vi "MS4_demo.vi"() -> ()   [LabVIEW 2012]
uses:
  States.ctl
  <vilib>/vision/Image Controls.llb/IMAQ Image.ctl
  <vilib>/httpClient/ClientHandle.ctl
  <vilib>/Platform/TimedLoop/XDataNode/timing_clust.ctl
  <vilib>/Platform/TimedLoop/XDataNode/nitl_modes.ctl
  <vilib>/Platform/TimedLoop/XDataNode/wakeup.ctl
  <vilib>/FPGAPlugInAG/sbRIO-9636/niLvFpga_Open_sbRIO-9636.vi
  <vilib>/rvi/interface/common/dynamic/niFpgaDynamicAddResources.vi
  Globals.vi
  <vilib>/Utility/error.llb/Error Cluster From Error Code.vi
  <vilib>/rvi/errors/niLvFpgaAdjustHostInterfaceError.vi
  <vilib>/FPGAPlugInAG/Dynamic/niLvFpga_Close_Dynamic.vi
  <vilib>/platform/TimedLoop/XDataNode/XDataNode.xnode
  <vilib>/rvi/interface/nirviOpenFPGA/nirviOpenFPGA.xnode
  FPGA Bitfiles/NIARC_FPGATarget_FPGACompile_e4XhunWUay0.lvbitx
  <vilib>/rvi/interface/nirviReadWriteControl/nirviReadWriteControl.xnode
  <vilib>/rvi/interface/nirviCloseFPGA/nirviCloseFPGA.xnode
  <vilib>/Platform/TimedLoop/XDataNode/XDNodeRunTimeDep.lvlib
  <vilib>/httpClient/LabVIEWHTTPClient.lvlib
  NiFpgaLv.dll
  <vilib>/rvi/interface/Simulation/niFpgaSimulationCallBeginRW.vi
panel:
  in  "WaypointWaypoints 2":dbl[][](array[numeric])
  in  "WaypointWaypoints":dbl[][](array[numeric])
  in  "Go to block?":bool=TRUE
  out "Arm State":enum16{"arm down", "push", "turn", "arm up"}(ring)
  out "Current \nState":T1(ring)
  in  "Claw deadband":dbl=0.05
  in  "Block Claw distance":dbl=0.25
  in  "stop":bool
  in  "Enable":bool
  in  "Block Mid Range":dbl=50.0
  in  "Block X-Offset":dbl=100.0
  # "Ignore Front ir"
  # "Heading"
  # "Forward Speed"
  # "Time (ms)"
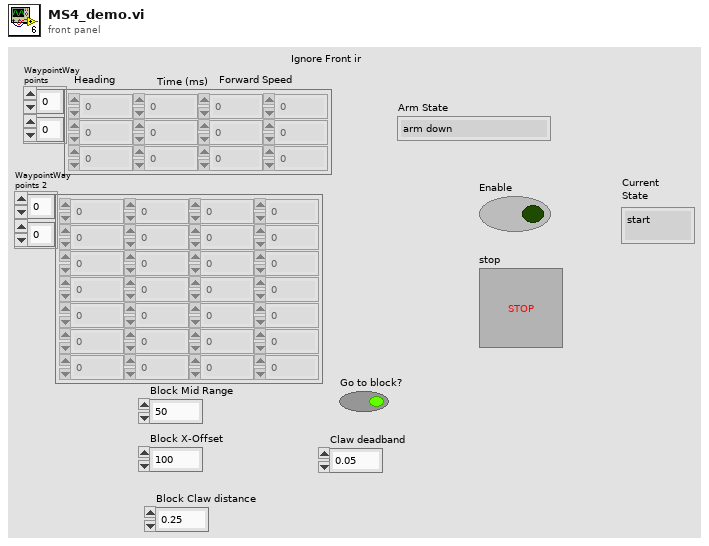
[diagram p1: front panel]
types:
  T1 = enum16{"start", "drive", "turning", "find block", "align block", "pickup"}
  T2 = cluster{"X Velocity (m/s)":dbl, "Y Velocity (m/s)":dbl, "Angular Velocity (rad/s)":dbl}
  T3 = typedef "IMAQ Image.ctl" = refnum<image>
  T4 = typedef "LabVIEWHTTPClient.lvlib/ClientHandle.ctl" = refnum<k1>
  T5 = cluster{"Camera":T3, "Track":T3, "client handle":T4}
  T6 = typedef "Image Type" = u32
  T7 = typedef "States.ctl" = enum16{"start", "drive", "turning", "find block", "align block", "pickup", "go home", "finish"}
  T8 = enum16{"wait", "open", "close", "lift", "lower", "pickup"}
  T9 = typedef "XDNodeRunTimeDep.lvlib/timing_clust.ctl" = cluster{"Expected End [f-1]":u64, "Actual End [f-1]":u64, "Finished Late? [f-1]":bool, "Expected End [i-1]":u64, "Actual End [i-1]":u64, "Finished Late? [i-1]":bool, "Expected Start [i]":u64, "Actual Start [i]":u64, "Expected Start [f]":u64, "Actual Start [f]":u64, "Source Name":string, "Structure Name":string, "Period":i64, "Deadline":i64, "Offset":i64, "Start":i64, "Priority":i32, "Timeout":i32, "Mode":T10, "Wakeup Reason":T11, "Error":errorcluster, "Source Type":string, "Secondary Source Type":string, "Global End Time":u64, "Global Start Time":u64, "Frame Duration":u64, "Iteration Duration":u64, "Assigned CPU":i32, "I/O Scan Engine Mode":u32}
  T10 = typedef "XDNodeRunTimeDep.lvlib/nitl_modes.ctl" = enum32{"No Change", "Process missed periods, maintain original phase", "Discard missed periods, maintain original phase", "Process missed periods, ignore original phase", "Discard missed periods, ignore original phase"}
  T11 = typedef "XDNodeRunTimeDep.lvlib/wakeup.ctl" = enum32{"Normal", "Aborted", "Asynchronous wakeup", "Timing source error", "Timed loop error", "Timeout"}
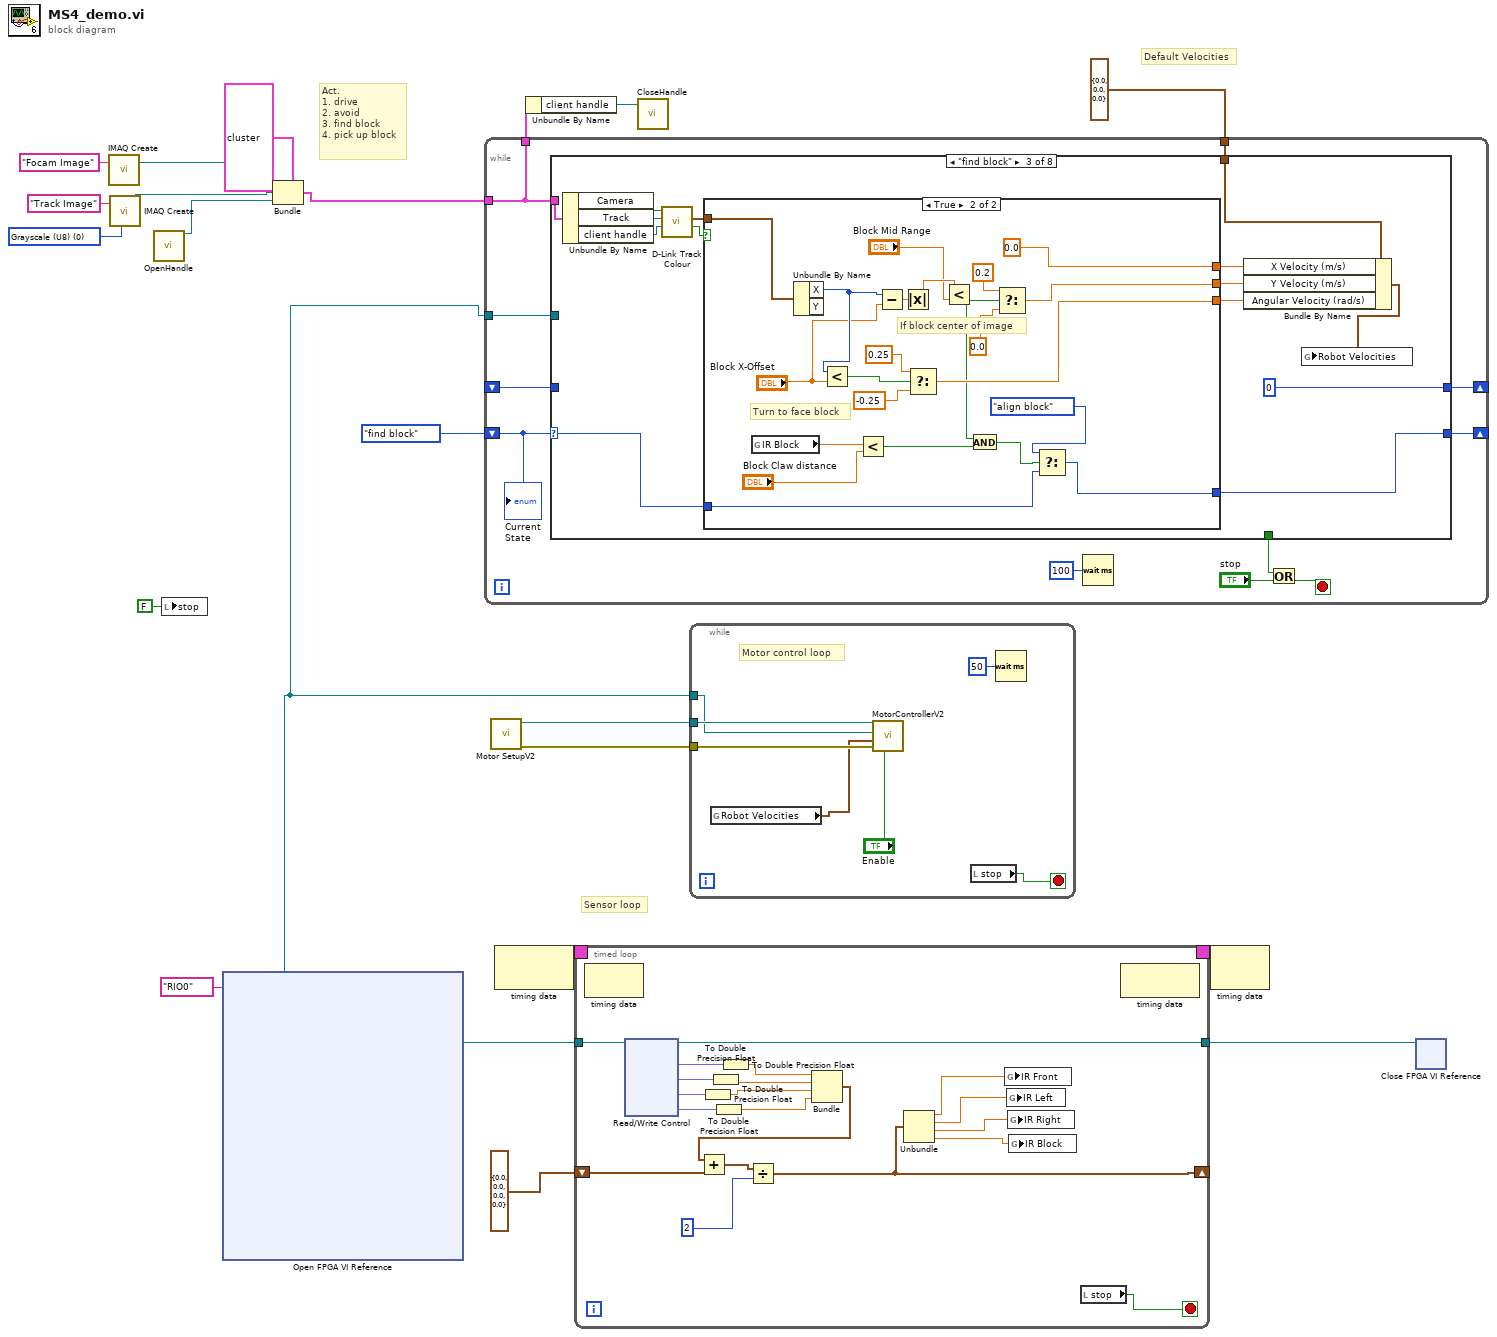
[diagram p0: block diagram]
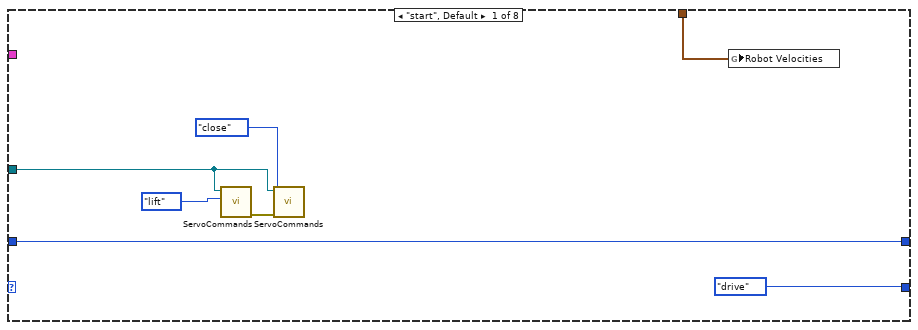
[diagram p2: hidden frame]
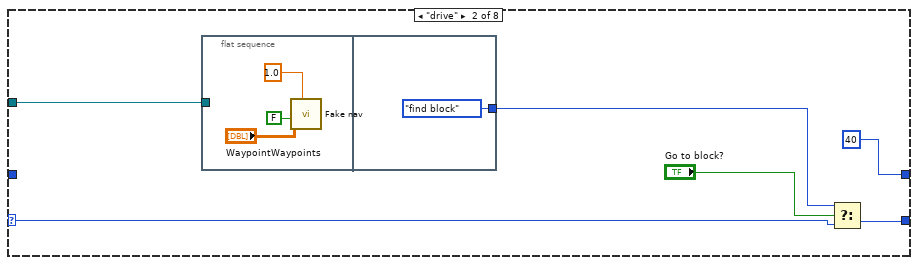
[diagram p3: hidden frame]
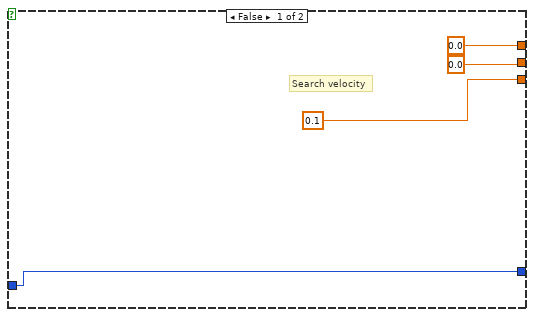
[diagram p4: hidden frame]
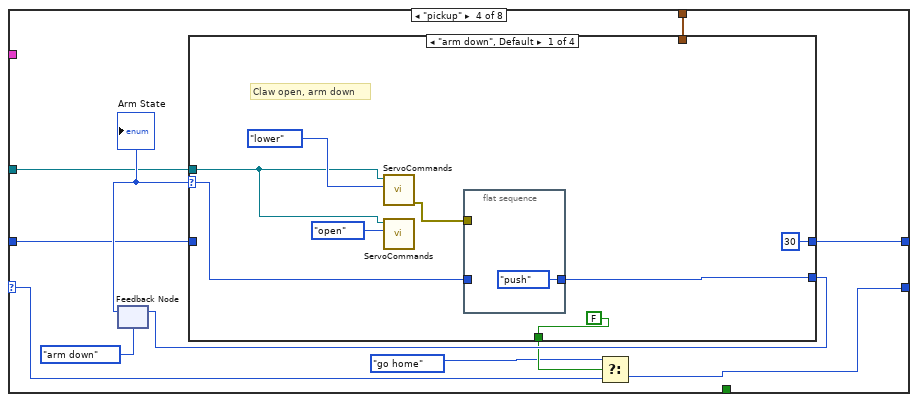
[diagram p5: hidden frame]
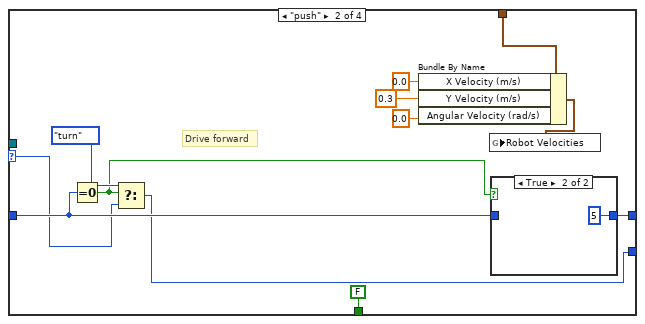
[diagram p6: hidden frame]
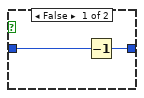
[diagram p7: hidden frame]
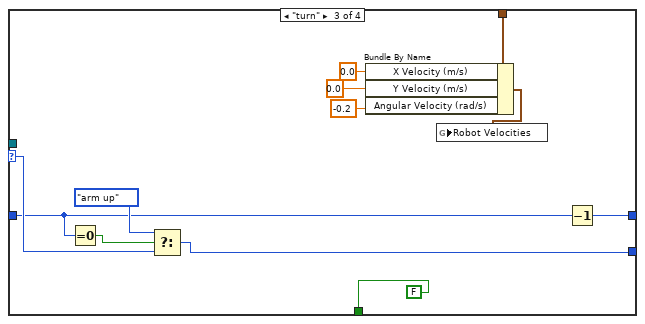
[diagram p8: hidden frame]
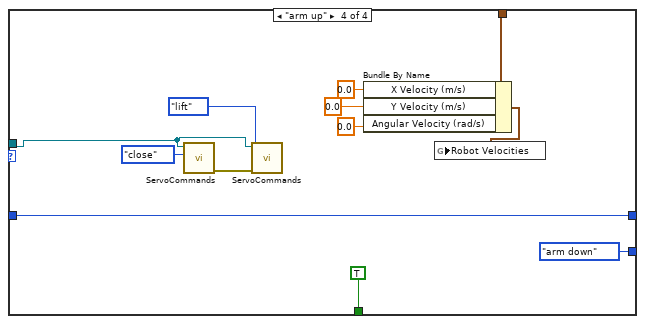
[diagram p9: hidden frame]
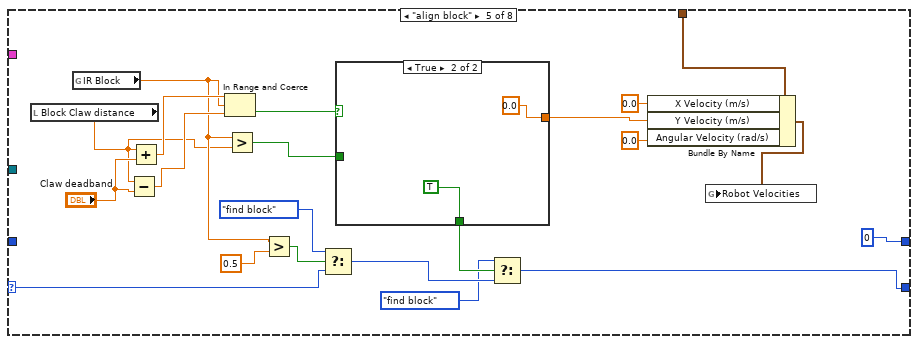
[diagram p10: hidden frame]
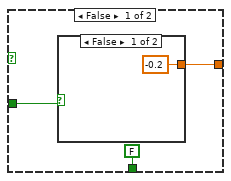
[diagram p11: hidden frame]
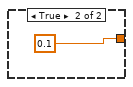
[diagram p12: hidden frame]
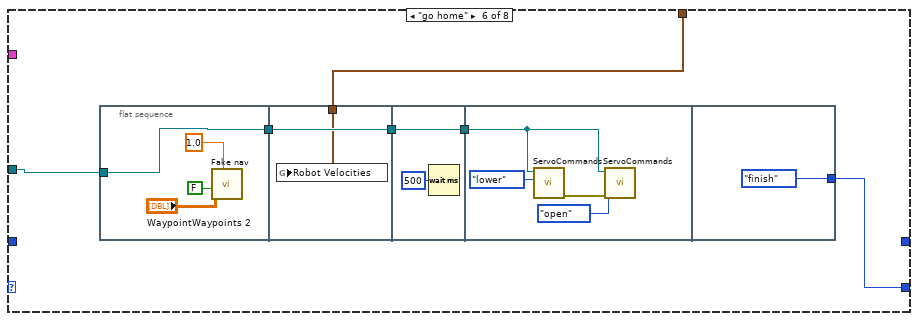
[diagram p13: hidden frame]
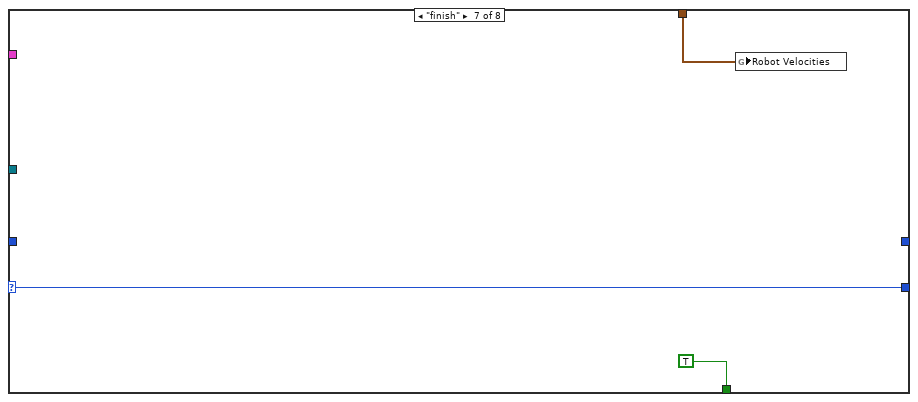
[diagram p14: hidden frame]
diagram:
  w14 = T6 0 items=["Grayscale (U8)", "Grayscale (I16)", "Grayscale (SGL)", "Complex (CSG)", "RGB (U32)", "HSL (U32)", "RGB (U64)", "Grayscale (U16)"] ("Image Type")
  # "Default Velocities"
  # "Sensor loop"
  # "Act.\n1. drive\n2. avoid\n3. find block\n4. pick up block"
  n1 = call "IMAQ Create"("Image Name"="Focam Image") -> ("New Image"=w12:T3)  [unwired: 4 in, 1 out]
  n2 = call "IMAQ Create"("Image Name"="Track Image", "Image Type"=w14) -> ("New Image"=w13:T3)  [unwired: 3 in, 1 out]
  n3 = call <vilib>:"OpenHandle.vi"() -> ("client handle out"=w3:T4)  [unwired: 14 in, 1 out]
  n4 = local write "stop"(FALSE ("stop")) -> ()
  n5 = xnode "Open FPGA VI Reference"("resource name"=tag "RIO0") -> ("FPGA VI Reference Out"=w4:refnum<k20>)  [unwired: 1 in, 1 out]
  n6 = Bundle(cluster=T5 {"Camera"=refnum, "Track"=refnum, "client handle"=refnum}, "Camera"=w12, "Track"=w13, "client handle"=w3) -> (w11:T5)
  n7 = while {
    shift-right: [w26] -> _
    shift-left: States."find block" -> [w25]
    shift-right: [w32] -> _
    shift-left: _ -> [w31]
    tunnel: w11 -> [w29]
    tunnel: [w29] -> w2
    tunnel: T2 {"X Velocity (m/s)"=0.0, "Y Velocity (m/s)"=0.0, "Angular Velocity (rad/s)"=0.0} ("Robot Velocities") -> [w27]
    tunnel: w4 -> [w24]
    stop <- w23 stop-if-true
    n8 = case shown="\"find block\"" w25 {
      selector: w25 -> [_ w41 w52 w93 w155 _ w198 w199]
      tunnel: [States."drive" w44 w51 w92 w152 w181 w198 w199] -> w26
      tunnel: [w39 40 0 w96 0 _ _ _] -> w32
      tunnel: w31 -> [w39 _ _ w97 _ _ _ _]
      tunnel: w29 -> [_ _ w62 _ _ _ _ _]
      tunnel: w27 -> [w34 _ w54 w95 w167 w180 w196 _]
      tunnel: w24 -> [w33 w42 _ w94 _ w182 _ _]
      tunnel: [_ _ _ _ _ _ TRUE _] -> w22
      frame "start", Default {
        n9 = call "ServoCommands.vi"("State"=T8."lift", "FPGA VI Reference In"=w33) -> ("error out"=w37:errorcluster)  [unwired: 9 in]
        n10 = call "ServoCommands.vi"("error in"=w37, "State"=T8."close", "FPGA VI Reference In"=w33) -> ()  [unwired: 8 in, 1 out]
        n11 = global write "Globals.vi" "Robot Velocities"(w34) -> ()
      }
      frame "drive" {
        n12 = flat-sequence {
          tunnel: w42 -> [_]
          tunnel: [States."find block"] -> w40
          frame #0 {
            n13 = call "Fake nav.vi"("Overall speed"=1.0, "Make start deg 0"=FALSE, "Array"="WaypointWaypoints") -> ()  [unwired: 9 in]
          }
          frame #1 {
          }
        }
        n14 = Select(t=w40, s="Go to block?", f=w41) -> (s? t:f=w44:T7)
      }
      frame "find block" {
        n15 = Unbundle By Name(w62) -> ("Camera"=w61:T3, "Track"=w60:T3, "client handle"=w50:T4)
        n16 = call "D-Link Track Colour.vi"("client handle"=w50, "Image Dst"=w60, "New Image"=w61) -> ("Object found?"=w53:bool, "Object Output"=w55:cluster{"X":i32, "Y":i32})  [unwired: 6 in, 1 out]
        n17 = case shown="True" w53 {
          tunnel: [0.0 ("X Velocity (m/s)") 0.0 ("X Velocity (m/s)")] -> w59
          tunnel: [0.1 ("f") w88] -> w58
          tunnel: [0.0 ("f") w84] -> w57
          tunnel: w55 -> [_ w78]
          tunnel: [w64 w71] -> w51
          tunnel: w52 -> [w64 w72]
          frame False {
            # "Search velocity"
          }
          frame True {
            # "Turn to face block"
            # "If block center of image"
            n18 = global read "Globals.vi" "IR Block"() -> (w77:dbl)
            n19 = Unbundle By Name(w78) -> ("X"=w81:i32)  [unwired: 1 out]
            n20 = Less?(x=w81, y="Block X-Offset") -> (x < y?=w85:bool)
            n21 = Less?(x=w77, y="Block Claw distance") -> (x < y?=w74:bool)
            n22 = Subtract(x=w81, y="Block X-Offset") -> (x-y=w79:dbl)
            n23 = Absolute Value(x=w79) -> (abs(x)=w70:dbl)
            n24 = Select(t=0.25, s=w85, f=-0.25) -> (s? t:f=w88:dbl)
            n25 = Less?(x=w70, y="Block Mid Range") -> (x < y?=w75:bool)
            n26 = And(x=w75, y=w74) -> (x .and. y?=w73:bool)
            n27 = Select(t=0.2, s=w75, f=0.0) -> (s? t:f=w84:dbl)
            n28 = Select(t=States."align block", s=w73, f=w72) -> (s? t:f=w71:T7)
          }
        }
        n29 = Bundle By Name(cluster=w54, "X Velocity (m/s)"=w59, "Y Velocity (m/s)"=w57, "Angular Velocity (rad/s)"=w58) -> (w56:T2)
        n30 = global write "Globals.vi" "Robot Velocities"(w56) -> ()
      }
      frame "pickup" {
        n31 = feedback #1(enum16{"arm down", "push", "turn", "arm up"}."arm down") -> (w98:enum16{"arm down", "push", "turn", "arm up"})
        "Arm State" <- w98
        n32 = case shown="\"arm down\", Default" w98 {
          selector: w98 -> [w104 w115 w136 _]
          tunnel: [w105 w114 w129 enum16{"arm down", "push", "turn", "arm up"}."arm down" ("t")] -> w100
          tunnel: w97 -> [_ w116 w127 w148]
          tunnel: [30 w117 w135 w148] -> w96
          tunnel: w95 -> [_ w118 w131 w143]
          tunnel: w94 -> [w101 _ _ w137]
          tunnel: [FALSE FALSE FALSE TRUE] -> w91
          frame "arm down", Default {
            # "Claw open, arm down"
            n33 = call "ServoCommands.vi"("State"=T8."lower", "FPGA VI Reference In"=w101) -> ("error out"=w103:errorcluster)  [unwired: 9 in]
            n34 = call "ServoCommands.vi"("State"=T8."open", "FPGA VI Reference In"=w101) -> ()  [unwired: 9 in, 1 out]
            n35 = flat-sequence {
              tunnel: [enum16{"arm down", "push", "turn", "arm up"}."push"] -> w105
              tunnel: w104 -> [_]
              tunnel: w103 -> [_]
              frame #0 {
              }
            }
          }
          frame "push" {
            # "Drive forward"
            n36 = Equal To 0?(x=w116) -> (x = 0?=w112:bool)
            n37 = Select(t=enum16{"arm down", "push", "turn", "arm up"}."turn", s=w112, f=w115) -> (s? t:f=w114:enum16{"arm down", "push", "turn", "arm up"})
            n38 = Bundle By Name(cluster=w118, "X Velocity (m/s)"=0.0, "Y Velocity (m/s)"=0.3, "Angular Velocity (rad/s)"=0.0) -> (w121:T2)
            n39 = global write "Globals.vi" "Robot Velocities"(w121) -> ()
            n40 = case shown="True" w112 {
              tunnel: [w123 5] -> w117
              tunnel: w116 -> [w122 _]
              frame False {
                n41 = Decrement(x=w122) -> (x-1=w123:i32)
              }
              frame True {
              }
            }
          }
          frame "turn" {
            n42 = Equal To 0?(x=w127) -> (x = 0?=w126:bool)
            n43 = Select(t=enum16{"arm down", "push", "turn", "arm up"}."arm up", s=w126, f=w136) -> (s? t:f=w129:enum16{"arm down", "push", "turn", "arm up"})
            n44 = Bundle By Name(cluster=w131, "X Velocity (m/s)"=0.0, "Y Velocity (m/s)"=0.0, "Angular Velocity (rad/s)"=-0.2) -> (w134:T2)
            n45 = global write "Globals.vi" "Robot Velocities"(w134) -> ()
            n46 = Decrement(x=w127) -> (x-1=w135:i32)
          }
          frame "arm up" {
            n47 = call "ServoCommands.vi"("State"=T8."close", "FPGA VI Reference In"=w137) -> ("error out"=w141:errorcluster)  [unwired: 9 in]
            n48 = call "ServoCommands.vi"("error in"=w141, "State"=T8."lift", "FPGA VI Reference In"=w137) -> ()  [unwired: 8 in, 1 out]
            n49 = Bundle By Name(cluster=w143, "X Velocity (m/s)"=0.0, "Y Velocity (m/s)"=0.0, "Angular Velocity (rad/s)"=0.0) -> (w147:T2)
            n50 = global write "Globals.vi" "Robot Velocities"(w147) -> ()
          }
        }
        n51 = feedback-in #1(w100) -> ()
        n52 = Select(t=States."go home", s=w91, f=w93) -> (s? t:f=w92:T7)
      }
      frame "align block" {
        n53 = local read "Block Claw distance"() -> (w151:dbl)
        n54 = global read "Globals.vi" "IR Block"() -> (w158:dbl)
        n55 = Subtract(x=w151, y="Claw deadband") -> (x-y=w160:dbl)
        n56 = Add(x=w151, y="Claw deadband") -> (x+y=w163:dbl)
        n57 = In Range and Coerce(upper limit=w163, x=w158, lower limit=w160) -> (In Range?=w162:bool)  [unwired: 1 out]
        n58 = Greater?(x=w158, y=w151) -> (0:w159:bool)
        n59 = Greater?(x=w158, y=0.5) -> (0:w156:bool)
        n60 = Select(t=States."find block", s=w156, f=w155) -> (s? t:f=w153:T7)
        n61 = case shown="True" w162 {
          tunnel: [w172 0.0 ("Y Velocity (m/s)")] -> w164
          tunnel: w159 -> [w171 _]
          tunnel: [FALSE TRUE] -> w154
          frame False {
            n62 = case shown="False" w171 {
              tunnel: [-0.2 ("Y Velocity (m/s)") 0.1 ("Y Velocity (m/s)")] -> w172
              frame False {
              }
              frame True {
              }
            }
          }
          frame True {
          }
        }
        n63 = Select(t=States."find block", s=w154, f=w153) -> (s? t:f=w152:T7)
        n64 = Bundle By Name(cluster=w167, "X Velocity (m/s)"=0.0, "Y Velocity (m/s)"=w164, "Angular Velocity (rad/s)"=0.0) -> (w168:T2)
        n65 = global write "Globals.vi" "Robot Velocities"(w168) -> ()
      }
      frame "go home" {
        n66 = flat-sequence {
          tunnel: w182 -> [w183]
          tunnel: [w183] -> w177
          tunnel: [w188] -> w179
          tunnel: w180 -> [w187]
          tunnel: w177 -> [w188]
          tunnel: w179 -> [w190]
          tunnel: [w190] -> w178
          tunnel: w178 -> [w191]
          tunnel: [States."finish"] -> w181
          frame #0 {
            n67 = call "Fake nav.vi"("Overall speed"=1.0, "Make start deg 0"=FALSE, "Array"="WaypointWaypoints 2") -> ()  [unwired: 9 in]
          }
          frame #1 {
            n68 = global write "Globals.vi" "Robot Velocities"(w187) -> ()
          }
          frame #2 {
            n69 = Wait (ms)(milliseconds to wait=u32 500) -> ()  [unwired: 1 out]
          }
          frame #3 {
            n70 = call "ServoCommands.vi"("State"=T8."lower", "FPGA VI Reference In"=w191) -> ("error out"=w192:errorcluster)  [unwired: 9 in]
            n71 = call "ServoCommands.vi"("error in"=w192, "State"=T8."open", "FPGA VI Reference In"=w191) -> ()  [unwired: 8 in, 1 out]
          }
          frame #4 {
          }
        }
      }
      frame "finish" {
        n72 = global write "Globals.vi" "Robot Velocities"(w196) -> ()
      }
      frame "turning" {
      }
    }
    n73 = Wait (ms)(milliseconds to wait=u32 100) -> ()  [unwired: 1 out]
    n74 = Or(x=w22, y="stop") -> (x .or. y?=w23:bool)
    "Current \nState" <- w25
  }
  n75 = call "Motor SetupV2.vi"() -> ("error out"=w20:errorcluster, "mecanum steering frame out"=w21:refnum<class "NI_Robotics_Mecanum Steering Frame.lvclass">)  [unwired: 10 in]
  n76 = node-c288() -> (w19:T9)  [unwired: 1 in]
  n77 = Unbundle By Name(w2) -> ("client handle"=w1:T4)
  n78 = timed-loop {
    timing: w19 -> [_]
    timing-out: [_] -> w18
    tunnel: w4 -> [w219]
    shift-right: [w208] -> _
    shift-left: cluster{dbl, dbl, dbl, dbl} {0.0, 0.0, 0.0, 0.0} -> [w212]
    tunnel: [w203] -> w7
    stop <- w204 stop-if-true
    n79 = node-c288() -> ()  [unwired: 1 in, 1 out]
    n80 = xnode "Read/Write Control"("FPGA VI Reference In"=w219) -> ("FPGA VI Reference Out"=w203:refnum<k20>, "IR 0"=w218:fxp<+/-,24,5>, "IR 1"=w217:fxp<+/-,24,5>, "IR 2"=w216:fxp<+/-,24,5>, "IR 3"=w202:fxp<+/-,24,5>)  [unwired: 1 in, 1 out]
    n81 = To Double Precision Float(number=w216) -> (double precision float=w213:dbl)
    n82 = To Double Precision Float(number=w217) -> (double precision float=w214:dbl)
    n83 = To Double Precision Float(number=w202) -> (double precision float=w201:dbl)
    n84 = To Double Precision Float(number=w218) -> (double precision float=w215:dbl)
    n85 = Bundle(w215, w214, w213, w201) -> (w211:cluster{dbl, dbl, dbl, dbl})  [unwired: 1 in]
    n86 = Add(x=w211, y=w212) -> (x+y=w210:cluster{dbl, dbl, dbl, dbl})
    n87 = Divide(x=w210, y=2) -> (x/y=w208:cluster{dbl, dbl, dbl, dbl})
    n88 = Unbundle(w208) -> (w207:dbl, w206:dbl, w205:dbl, w200:dbl)
    n89 = global write "Globals.vi" "IR Front"(w207) -> ()
    n90 = global write "Globals.vi" "IR Left"(w206) -> ()
    n91 = global write "Globals.vi" "IR Right"(w205) -> ()
    n92 = global write "Globals.vi" "IR Block"(w200) -> ()
    n93 = local read "stop"() -> (w204:bool)
    n94 = node-c288() -> ()  [unwired: 1 in, 1 out]
  }
  n95 = call <vilib>:"CloseHandle.vi"("client handle"=w1) -> ()  [unwired: 14 in, 1 out]
  n96 = while {
    tunnel: w21 -> [w228]
    tunnel: w20 -> [w227]
    tunnel: w4 -> [w226]
    stop <- w222 stop-if-true
    # "Motor control loop"
    n97 = global read "Globals.vi" "Robot Velocities"() -> (w225:T2)
    n98 = call "MotorControllerV2.vi"("Enable"="Enable", "error in"=w227, "Robot Velocities"=w225, "FPGA VI Reference In"=w226, "mecanum steering frame in"=w228) -> ()  [unwired: 5 in, 2 out]
    n99 = local read "stop"() -> (w222:bool)
    n100 = Wait (ms)(milliseconds to wait=u32 50) -> ()  [unwired: 1 out]
  }
  n101 = node-c288(w18) -> ()  [unwired: 1 out]
  n102 = xnode "Close FPGA VI Reference"("FPGA VI Reference In"=w7) -> ()  [unwired: 1 in, 1 out]
